vi "Connect DVR Terminals.vi"(8 "error in (no error)":errorcluster, 11 "DVR VI Path":path=path "D:/GitHub/LabVIEW/SLL/Tools/Class DVR API Generator/Test/Test VI.vi") -> (0 "error out":errorcluster)   [LabVIEW 2016, in "SLL Scripting.lvlib" / "SLL Class DVR API Generator.lvlib"]
uses:
  SLL Class DVR API Generator.lvlib
  <vilib>/Utility/traverseref.llb/TRef TravTarget.ctl
  <vilib>/Utility/traverseref.llb/VI Scripting - Traverse.lvlib
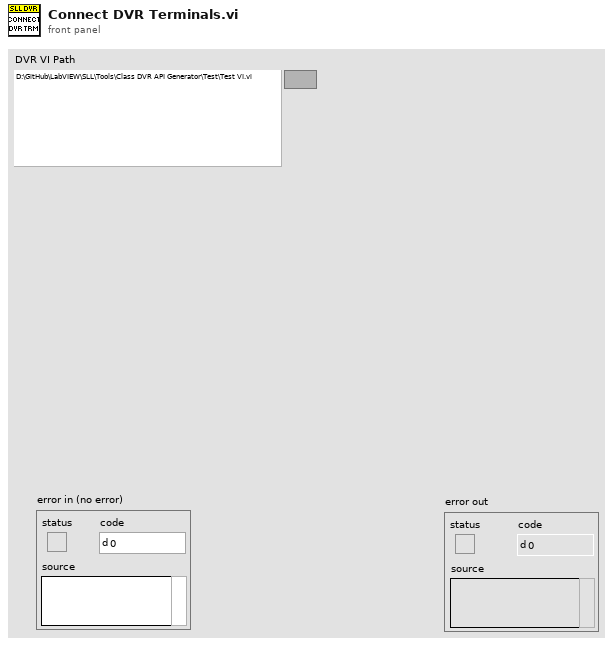
[diagram p1: front panel]
types:
  T1 = typedef "TRef TravTarget.ctl" = enum16{"FP", "BD", "Other"}
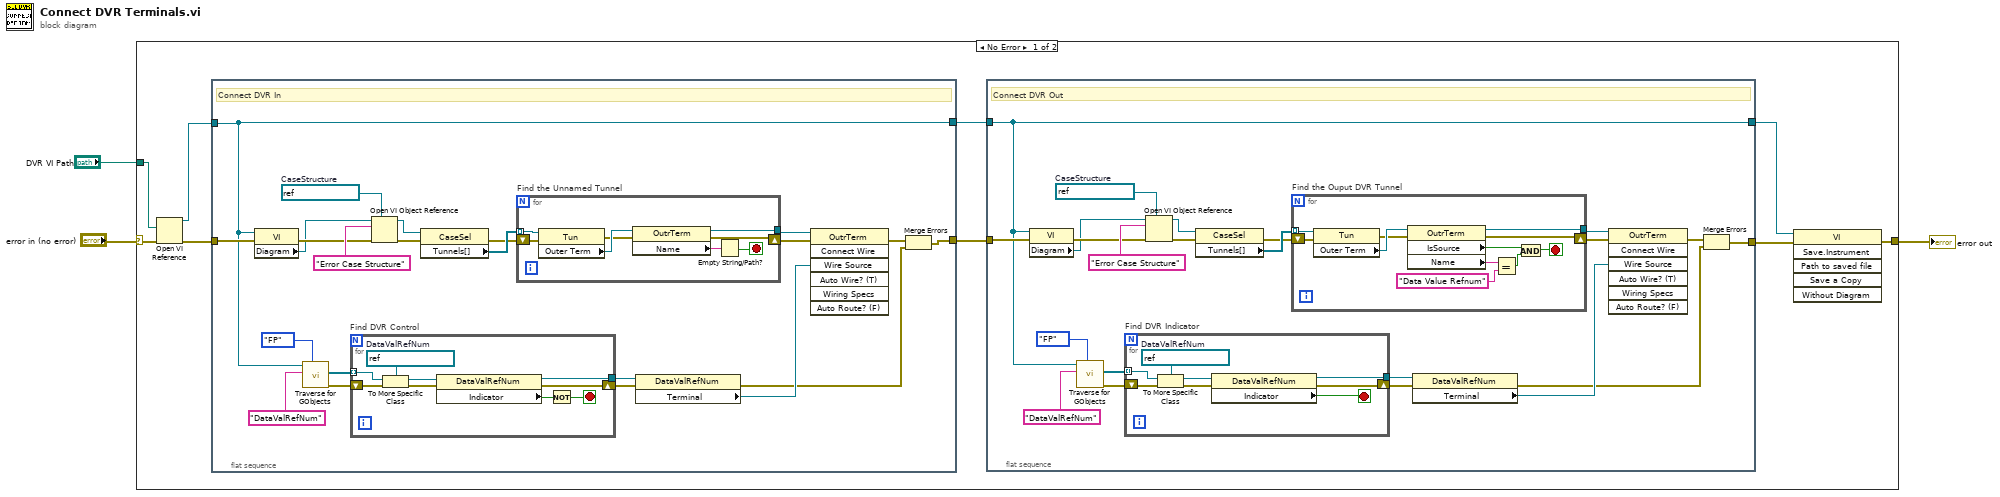
[diagram p0: block diagram]
diagram:
  n1 = case shown="No Error" "error in (no error)" {
    selector: "error in (no error)" -> [w12 w93]
    tunnel: [w10 w93] -> w2
    tunnel: "DVR VI Path" -> [w11 _]
    frame No Error {
      n2 = Open VI Reference(vi path=w11, error in (no error)=w12) -> (vi reference=w9:refnum<vi>, error out=w8:errorcluster)  [unwired: 4 in]
      n3 = flat-sequence {
        tunnel: w8 -> [w71]
        tunnel: w9 -> [w58]
        tunnel: [w59] -> w7
        tunnel: [w58] -> w6
        frame #0 {
          w65 = refnum<vi> refnum  # CaseStructure
          # "Connect DVR In"
          n4 = property class="VI"(reference=w58, error in=w71) -> (error out=w69:errorcluster, "Diagram"=w68:refnum<vi>)  [unwired: 1 out]
          n5 = call <vilib>:"Traverse for GObjects.vi"("Traverse Target"=TRef_TravTarget."FP", "Class Name"="DataValRefNum", "VI Refnum"=w58) -> ("error out"=w73:errorcluster, "References"=w72:refnum<vi>[])  [unwired: 5 in, 2 out]
          n6 = for "Find DVR Control" {
            shift-right: [w88] -> w56
            shift-left: w73 -> [w92]
            tunnel: w72 -> [w90] mode=indexing
            tunnel: [w84] -> w57
            stop <- w85 stop-if-true
            w89 = refnum<vi> refnum  # DataValRefNum
            n7 = To More Specific Class(target class=w89, reference=w90, error in=w92) -> (specific class reference=w87:refnum<vi>, error out=w91:errorcluster)
            n8 = property class="DataValRefNum"(reference=w87, error in=w91) -> (reference out=w84:refnum<vi>, error out=w88:errorcluster, "Indicator"=w86:bool)
            n9 = Not(x=w86) -> (.not. x?=w85:bool)
          }
          n10 = Open VI Object Reference(7:w65, 8:w69, 10:"Error Case Structure" ("name/order"), 11:w68) -> (0:w66:errorcluster, 3:w64:refnum<vi>)
          n11 = property class="CaseSel"(reference=w64, error in=w66) -> (error out=w63:errorcluster, "Tunnels[]"=w67:refnum<vi>[])  [unwired: 1 out]
          n12 = for "Find the Unnamed Tunnel" {
            tunnel: w67 -> [w83] mode=indexing
            shift-right: [w80] -> w62
            shift-left: w63 -> [w81]
            tunnel: [w76] -> w61
            stop <- w77 stop-if-true
            n13 = property class="Tun"(reference=w83, error in=w81) -> (error out=w79:errorcluster, "Outer Term"=w82:refnum<vi>)  [unwired: 1 out]
            n14 = property class="OutrTerm"(reference=w82, error in=w79) -> (reference out=w76:refnum<vi>, error out=w80:errorcluster, "Name"=w78:string)
            n15 = Empty String/Path?(string/path=w78) -> (empty?=w77:bool)
          }
          n16 = property class="DataValRefNum"(reference=w57, error in=w56) -> (error out=w54:errorcluster, "Terminal"=w55:refnum<vi>)  [unwired: 1 out]
          n17 = invoke class="OutrTerm" method="Connect Wire"(reference=w61, error in=w62, "Wire Source"=w55) -> (error out=w60:errorcluster)  [unwired: 4 in, 6 out]
          n18 = Merge Errors(w60, w54) -> (w59:errorcluster)
        }
      }
      n19 = flat-sequence {
        tunnel: w7 -> [w30]
        tunnel: w6 -> [w17]
        tunnel: [w18] -> w5
        tunnel: [w17] -> w4
        frame #0 {
          w24 = refnum<vi> refnum  # CaseStructure
          # "Connect DVR Out"
          n20 = property class="VI"(reference=w17, error in=w30) -> (error out=w28:errorcluster, "Diagram"=w27:refnum<vi>)  [unwired: 1 out]
          n21 = call <vilib>:"Traverse for GObjects.vi"("Traverse Target"=TRef_TravTarget."FP", "Class Name"="DataValRefNum", "VI Refnum"=w17) -> ("error out"=w32:errorcluster, "References"=w31:refnum<vi>[])  [unwired: 5 in, 2 out]
          n22 = for "Find DVR Indicator" {
            shift-right: [w49] -> w15
            shift-left: w32 -> [w53]
            tunnel: w31 -> [w51] mode=indexing
            tunnel: [w47] -> w16
            stop <- w46 stop-if-true
            w50 = refnum<vi> refnum  # DataValRefNum
            n23 = To More Specific Class(target class=w50, reference=w51, error in=w53) -> (specific class reference=w48:refnum<vi>, error out=w52:errorcluster)
            n24 = property class="DataValRefNum"(reference=w48, error in=w52) -> (reference out=w47:refnum<vi>, error out=w49:errorcluster, "Indicator"=w46:bool)
          }
          n25 = Open VI Object Reference(7:w24, 8:w28, 10:"Error Case Structure" ("name/order"), 11:w27) -> (0:w25:errorcluster, 3:w23:refnum<vi>)
          n26 = property class="CaseSel"(reference=w23, error in=w25) -> (error out=w22:errorcluster, "Tunnels[]"=w26:refnum<vi>[])  [unwired: 1 out]
          n27 = for "Find the Ouput DVR Tunnel" {
            tunnel: w26 -> [w45] mode=indexing
            shift-right: [w42] -> w21
            shift-left: w22 -> [w43]
            tunnel: [w40] -> w20
            stop <- w35 stop-if-true
            n28 = property class="Tun"(reference=w45, error in=w43) -> (error out=w41:errorcluster, "Outer Term"=w44:refnum<vi>)  [unwired: 1 out]
            n29 = property class="OutrTerm"(reference=w44, error in=w41) -> (reference out=w40:refnum<vi>, error out=w42:errorcluster, "IsSource"=w36:bool, "Name"=w39:string)
            n30 = Equal?(x=w39, y="Data Value Refnum") -> (x = y?=w37:bool)
            n31 = And(x=w36, y=w37) -> (x .and. y?=w35:bool)
          }
          n32 = property class="DataValRefNum"(reference=w16, error in=w15) -> (error out=w13:errorcluster, "Terminal"=w14:refnum<vi>)  [unwired: 1 out]
          n33 = invoke class="OutrTerm" method="Connect Wire"(reference=w20, error in=w21, "Wire Source"=w14) -> (error out=w19:errorcluster)  [unwired: 4 in, 6 out]
          n34 = Merge Errors(w19, w13) -> (w18:errorcluster)
        }
      }
      n35 = invoke class="VI" method="Save.Instrument"(reference=w4, error in=w5) -> (error out=w10:errorcluster)  [unwired: 4 in, 5 out]
    }
    frame Error {
    }
  }
  "error out" <- w2
